vi "Storage Line Construct.vi"() -> ()   [LabVIEW 2015]
panel:
  out "Cluster":T1
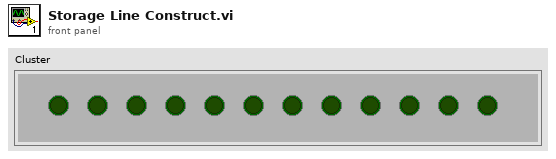
[diagram p1: front panel]
types:
  T1 = cluster{"Storage 1":bool, "Storage 2":bool, "Storage 3":bool, "Storage 4":bool, "Storage 5":bool, "Storage 6":bool, "Storage 7":bool, "Storage 8":bool, "Storage 9":bool, "Storage 10":bool, "Storage 11":bool, "Storage 12":bool}
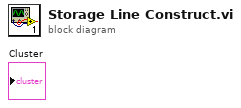
[diagram p0: block diagram]
diagram:
